vi "teste_pegar_boneco.vi"   [LabVIEW 2016]
uses:
  <vilib>/NXT/Subs/LVHSConnector.ctl
  <vilib>/NXT/LegoClasses/BrickReference/BrickReference.lvclass
  <vilib>/NXT/Block Support/NXT_OutputPort.ctl
  <vilib>/NXT/NXTIO Xnodes/NXTIONodeSubVIs/NXTMoveMotors.vi
  <vilib>/NXT/Dual Mode Library/Waits/Wait_Num.vi
  <vilib>/NXT/NXTIO Xnodes/NXTIONodeSubVIs/NXTStopMotors.vi
  <vilib>/NXT/NXTIO Xnodes/AddressXNode/NXTIOAddress.xnode
  <vilib>/NXT/NXTIO Xnodes/NXTIOXNode/NXTIO.xnode
types:
  T1 = typedef "LVHSConnector.ctl" = refnum<class "BrickReference.lvclass">
  T2 = typedef "NXT_OutputPort.ctl" = u8
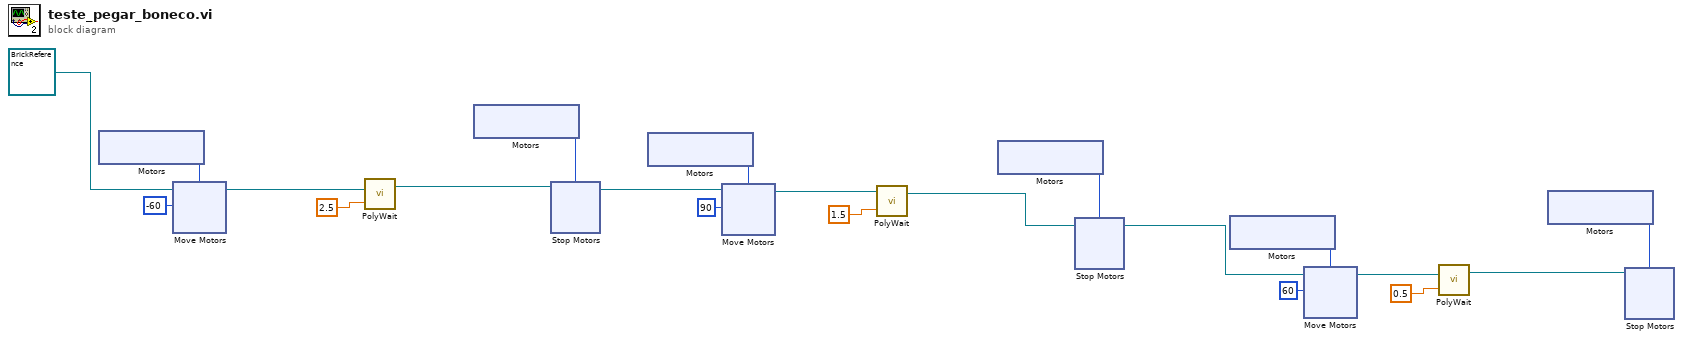
[diagram p0: block diagram]
diagram:
  n1 = xnode "Motors"() -> ("Motor"=w20:T2)
  n2 = xnode "Move Motors"("Power/Speed 1"=i8 -60, "Motors"=w20, "NXT/EV3"=T1 refnum ("ROBOIME 2")) -> ("NXT/EV3"=w19:T1)
  n3 = call-poly <vilib>:"PolyWait.vi"("Time (1 sec)"=sgl 2.5, "NXT/EV3"=w19) -> ("NXT/EV3"=w17:T1)  [unwired: 2 in]
  n4 = xnode "Motors"() -> ("Motor"=w16:T2)
  n5 = xnode "Stop Motors"("Motors"=w16, "NXT/EV3"=w17) -> ("NXT/EV3"=w15:T1)
  n6 = xnode "Motors"() -> ("Motor"=w13:T2)
  n7 = xnode "Move Motors"("Power/Speed 1"=i8 90, "Motors"=w13, "NXT/EV3"=w15) -> ("NXT/EV3"=w10:T1)
  n8 = call-poly <vilib>:"PolyWait.vi"("Time (1 sec)"=sgl 1.5, "NXT/EV3"=w10) -> ("NXT/EV3"=w8:T1)  [unwired: 2 in]
  n9 = xnode "Motors"() -> ("Motor"=w9:T2)
  n10 = xnode "Stop Motors"("Motors"=w9, "NXT/EV3"=w8) -> ("NXT/EV3"=w5:T1)
  n11 = xnode "Motors"() -> ("Motor"=w7:T2)
  n12 = xnode "Move Motors"("Power/Speed 1"=i8 60, "Motors"=w7, "NXT/EV3"=w5) -> ("NXT/EV3"=w1:T1)
  n13 = call-poly <vilib>:"PolyWait.vi"("Time (1 sec)"=sgl 0.5, "NXT/EV3"=w1) -> ("NXT/EV3"=w4:T1)  [unwired: 2 in]
  n14 = xnode "Motors"() -> ("Motor"=w3:T2)
  n15 = xnode "Stop Motors"("Motors"=w3, "NXT/EV3"=w4) -> ()  [unwired: 1 out]
